vi "Update_Install_Path.vi"(8 "error in (no error)":errorcluster, 10 "destName/Path":string, 11 "absFolder in":refnum<class "absFolder.lvclass">) -> (0 "error out":errorcluster, 3 "absFolder out":refnum<class "absFolder.lvclass">)   [LabVIEW 2020, in "absFolder.lvclass"]
uses:
  <vilib>/AppBuilder/IB_Classes/Destination/absFolder/absFolder.lvclass
  <vilib>/AppBuilder/IB_Classes/Destination/absFolder/absFolder.lvclass/absFolder.ctl
  <vilib>/AppBuilder/IB_Classes/Destination/IB_Destination.lvclass
  e:/builds/penguin/labview/branches/2020/dev/dist/vi.lib/AppBuilder/IB_Classes/Destination/IB_Destination.lvclass
  e:/builds/penguin/labview/branches/2020/dev/dist/vi.lib/AppBuilder/IB_Classes/Destination/absFolder/absFolder.lvclass
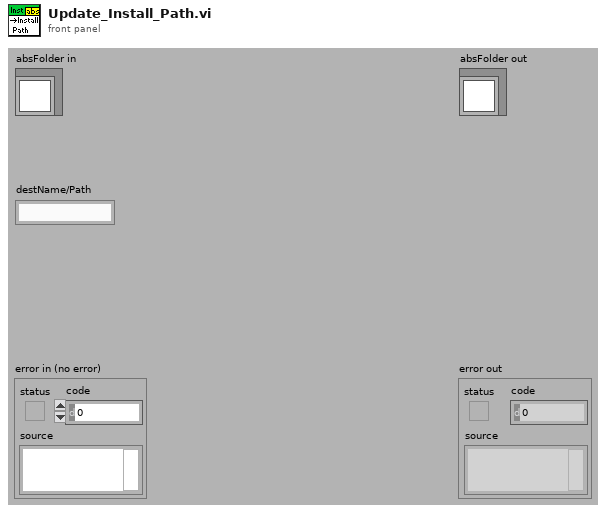
[diagram p1: front panel]
types:
  T1 = typedef "IB_Destination.ctl" = cluster{"name":string, "unlock":bool, "parentTag":string, "destTag":string, "eng_installPath":string}
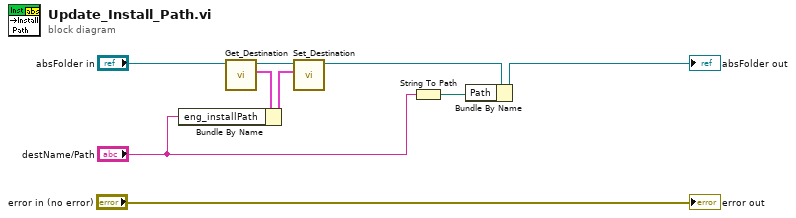
[diagram p0: block diagram]
diagram:
  n1 = call <vilib>:"Get_Destination.vi"("IB_Destination in"="absFolder in") -> ("data"=w8:T1, "IB_Destination out"=w9:refnum<class "absFolder.lvclass">)  [unwired: 1 in, 8 out]
  n2 = Bundle By Name(cluster=w8, "eng_installPath"="destName/Path") -> (w7:T1)
  n3 = call <vilib>:"Set_Destination.vi"("data"=w7, "IB_Destination in"=w9) -> ("IB_Destination out"=w4:refnum<class "absFolder.lvclass">)  [unwired: 1 in, 8 out]
  n4 = String To Path(string="destName/Path") -> (path=w1:path)
  n5 = Bundle By Name(cluster=w4, "Path"=w1) -> (→"absFolder out":refnum<class "absFolder.lvclass">)
  "error out" <- "error in (no error)"
